vi "OEE_read_config_files_to_fgv.vi"(8 "error_in":errorcluster, 11 "all_config_info_in":T1) -> (0 "error_out":errorcluster, 3 "all_config_info_out":T1)   [LabVIEW 2019]
uses:
  typedef/OEE_all_config_info.ctl
  typedef/OEE_main_ini_file.ctl
  queues/typedef/OEE_queue_refnums.ctl
  queues/typedef/OEE_MAIN_queue_element.ctl
  MAIN/OEE_MAIN_sequence_state.ctl
  queues/typedef/OEE_SCREEN_1_queue_element.ctl
  SCREEN_1/OEE_SCREEN_1_sequence_state.ctl
  queues/typedef/OEE_SCREEN_2_queue_element.ctl
  SCREEN_2/OEE_SCREEN_2_sequence_state.ctl
  queues/typedef/OEE_PULSE_queue_element.ctl
  PULSE/OEE_PULSE_sequence_state.ctl
  queues/typedef/OEE_GRAPH_TOGGLE_TIMER_queue_element.ctl
  SCREEN_2/GRAPH_TOGGLE_TIMER/OEE_GRAPH_TOGGLE_TIMER_sequence_state.ctl
  FGV/config_info/FGV_OEE_config_info.ctl
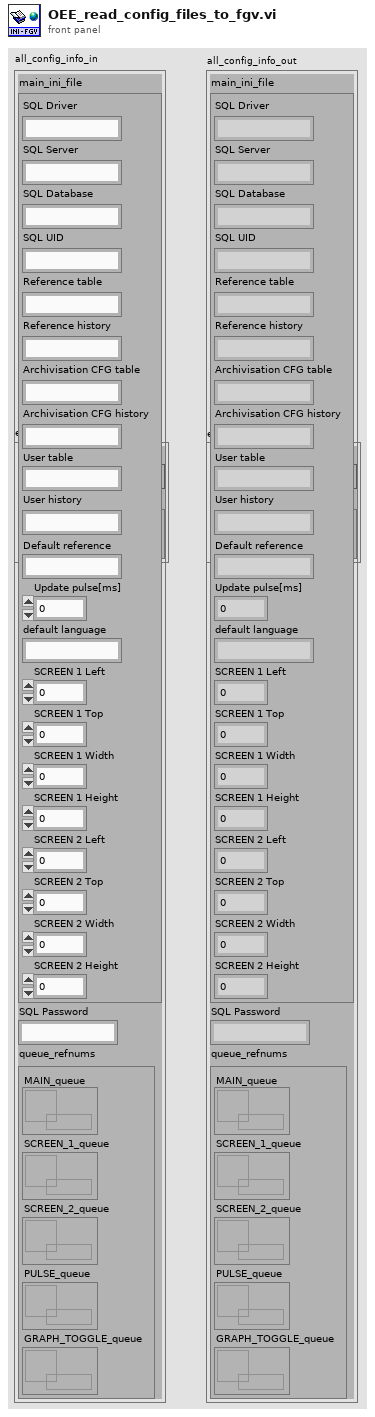
[diagram p1: front panel]
types:
  T1 = typedef "OEE_all_config_info.ctl" = cluster{"main_ini_file":T2, "SQL Password":string, "queue_refnums":T3}
  T2 = typedef "OEE_main_ini_file.ctl" = cluster{"SQL Driver":string, "SQL Server":string, "SQL Database":string, "SQL UID":string, "Reference table":string, "Reference history":string, "Archivisation CFG table":string, "Archivisation CFG history":string, "User table":string, "User history":string, "Default reference":string, "Update pulse[ms]":i32, "default language":string, "SCREEN 1 Left":i16, "SCREEN 1 Top":i16, "SCREEN 1 Width":i16, "SCREEN 1 Height":i16, "SCREEN 2 Left":i16, "SCREEN 2 Top":i16, "SCREEN 2 Width":i16, "SCREEN 2 Height":i16}
  T3 = typedef "OEE_queue_refnums.ctl" = cluster{"MAIN_queue":refnum<queue>, "SCREEN_1_queue":refnum<queue>, "SCREEN_2_queue":refnum<queue>, "PULSE_queue":refnum<queue>, "GRAPH_TOGGLE_queue":refnum<queue>}
  T4 = typedef "FGV_OEE_config_info.ctl" = enum16{"initialize", "set", "get"}
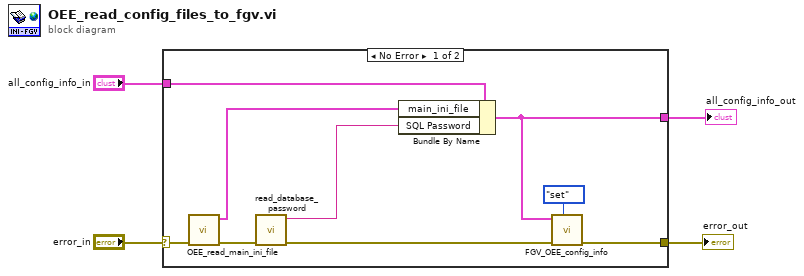
[diagram p0: block diagram]
diagram:
  n1 = case shown="No Error" "error_in" {
    selector: "error_in" -> [w13 w15]
    tunnel: [w11 w15] -> w4
    tunnel: [w5 w14] -> w1
    tunnel: "all_config_info_in" -> [w10 w14]
    frame No Error {
      n2 = call "OEE_read_main_ini_file.vi"("error_in"=w13) -> ("error_out"=w9:errorcluster, "main_ini_file_out"=w6:T2)  [unwired: 7 in, 2 out]
      n3 = call "read_database_password.vi"("error_in"=w9) -> ("error_out"=w8:errorcluster, "database_password"=w7:string)  [unwired: 8 in]
      n4 = Bundle By Name(cluster=w10, "main_ini_file"=w6, "SQL Password"=w7) -> (w5:T1)
      n5 = call "FGV_OEE_config_info.vi"("options"=FGV_OEE_config_info."set", "error_in"=w8, "all_config_info_in"=w5) -> ("error_out"=w11:errorcluster)  [unwired: 7 in, 1 out]
    }
    frame Error {
    }
  }
  "error_out" <- w4
  "all_config_info_out" <- w1
